vi "Ipvn.vi"(1 "Iscn":dbl, 2 "Rs":dbl, 3 "Rp":dbl) -> (0 "Ipvn":dbl)   [LabVIEW 2016]
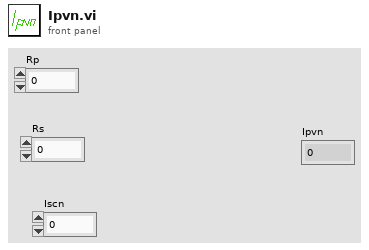
[diagram p1: front panel]
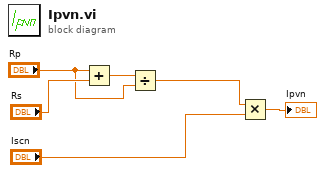
[diagram p0: block diagram]
diagram:
  n1 = Add(x="Rp", y="Rs") -> (x+y=w5:dbl)
  n2 = Divide(x=w5, y="Rp") -> (x/y=w2:dbl)
  n3 = Multiply(x=w2, y="Iscn") -> (x*y=→"Ipvn":dbl)
